vi "Global GUIDs.vi"() -> ()   [LabVIEW 2015, in "Waveform Data Logger Shared.lvlib"]
uses:
  Waveform Data Logger Shared.lvlib
panel:
  in  "File Status":string="09B4C131-8B17-4783-89F0-ADA0D62A49B5"
  in  "Missed Samples":string="312422B9-1139-4EBC-94A0-F12CDE6EA8BF"
  in  "TDMS Error Code":string="055BD3EF-920F-47E9-818D-A5F1CAC04AB2"
  in  "DAQ Wfm":string="E0B9F5F5-17A2-46AF-8A60-D4B1A03C728E"
  in  "Logging Group":string="50203BE4-F1CF-4448-B6B5-1A70CE9F8A31"
  in  "File":string="DFFDB176-AB83-475E-94F4-749A89FBE3A1"
  in  "Start New File":string="95DF4880-8622-4437-A2B8-4A33619268EB"
  in  "Logging Enabled":string="C7CD7F5B-9AA0-449F-B96F-5A38696788F1"
  in  "Root":string="BC5AD968-EDEC-4A39-A53C-A70162F6F464"
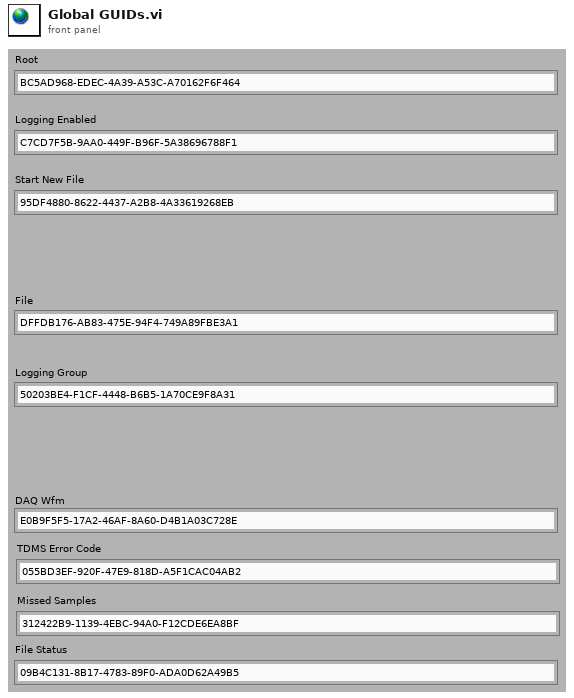
[diagram p1: front panel]
diagram:
